vi "Config Unflatten.vi"(8 "error in (no error)":errorcluster, 10 "Raw Config":string, 11 "launcher in":refnum<class "launcher.lvclass">) -> (0 "error out":errorcluster, 1 "Modified?":bool, 3 "launcher out":refnum<class "launcher.lvclass">)   [LabVIEW 2021, in "launcher.lvclass"]
uses:
  launcher.lvclass
  launcher.lvclass/launcher.ctl
  5cad098a-3cfd-4683-b1d7-f77832a71d5c.vi
  9da31e51-d9e1-4e00-992a-b5057d501661.vi
  c0ef7aaf-9b39-40b0-914c-f7984f3f44cf.vi
  b278cc91-79ab-40b4-b454-5ce35c9e2d2c.vi
  Accessors/Read _PARMS.vi
  Accessors/Write _PARMS.vi
  <vilib>/JDP Science/JSONtext/JSON text to Variant.vi
  <vilib>/JDP Science/JSONtext/LVClass Serializer/JSONtext LVClass Serializer.lvclass
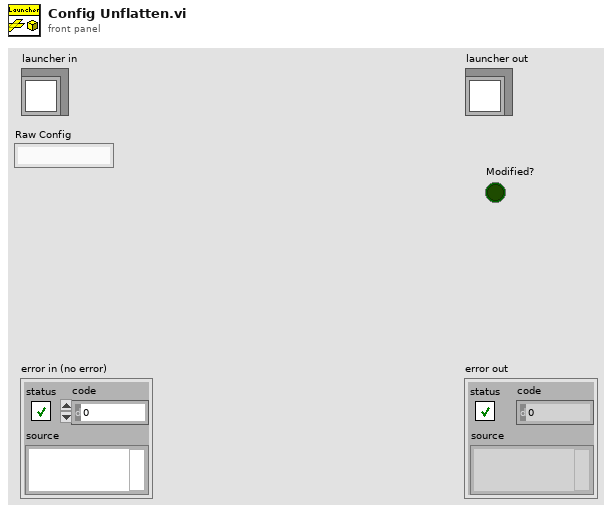
[diagram p1: front panel]
types:
  T1 = typedef "launcher.lvclass/_PARMS.ctl" = cluster{"ch_alias":string[], "ch_units":string[], "Modules to Launch":T2[]}
  T2 = typedef "Module.lvclass/Launch Module Typdef.ctl" = cluster{"Module":string, "Parameters":T3}
  T3 = typedef "Module.lvclass/Launch Module Parms.ctl" = cluster{"Name":string, "Arguments":string[], "Show FP?":bool}
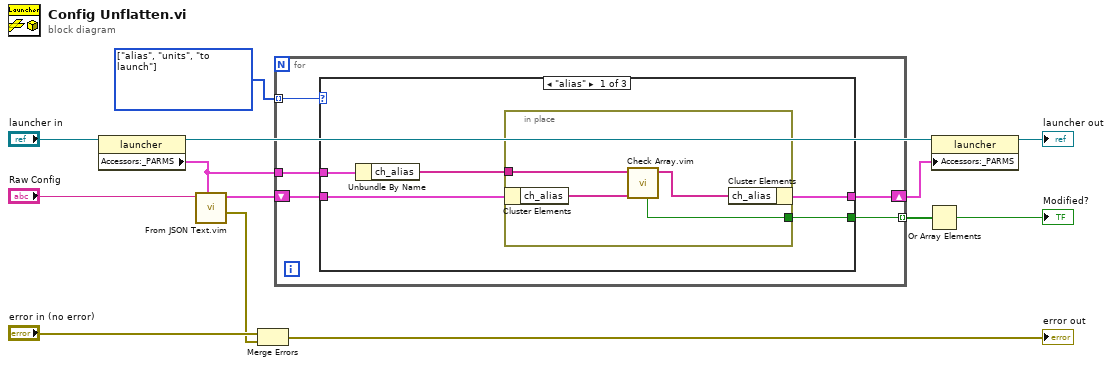
[diagram p0: block diagram]
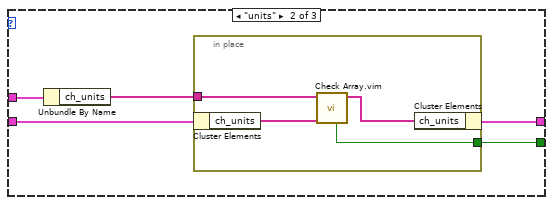
[diagram p2: hidden frame]
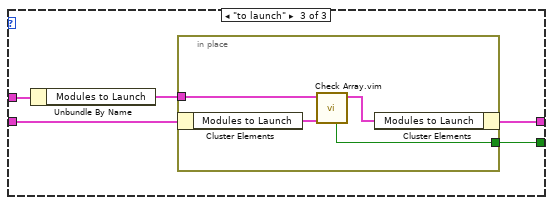
[diagram p3: hidden frame]
diagram:
  w7 = enum16{"alias", "units", "to launch"}[] [enum."alias", enum."units", enum."to launch"] items=["alias", "units", "to launch"]
  n1 = property class="launcher"(reference="launcher in") -> (reference out=w3:refnum<class "launcher.lvclass">, "Accessors:_PARMS"=w5:T1)  [unwired: 1 in, 1 out]
  n2 = call "From JSON Text.vim"("Data Type and Default Value"=w5, "JSON"="Raw Config") -> ("error out"=w9:errorcluster, "Data out"=w8:T1)  [unwired: 8 in]
  n3 = Merge Errors("error in (no error)", w9) -> (→"error out":errorcluster)
  n4 = for {
    shift-right: [w14] -> w2
    shift-left: w8 -> [w16]
    tunnel: w7 -> [w18] mode=indexing
    tunnel: w5 -> [w17]
    tunnel: [w15] -> w6 mode=indexing
    n5 = case shown="\"alias\"" w18 {
      tunnel: w17 -> [w22 w31 w40]
      tunnel: w16 -> [w21 w30 w39]
      tunnel: [w23 w32 w41] -> w15
      tunnel: [w19 w28 w37] -> w14
      frame "alias" {
        n6 = Unbundle By Name(w22) -> ("ch_alias"=w20:string[])
        n7 = in-place {
          in-place-border: [w26] -> w23
          in-place-border: w20 -> [w24]
          n8 = in-place-cluster #1(w21) -> ("ch_alias"=w25:string[])
          n9 = call "Check Array.vim"("Value in"=w25, "Default Value"=w24) -> ("Value out"=w27:string[], "Modified?"=w26:bool)  [unwired: 8 in]
          n10 = in-place-cluster #1("ch_alias"=w27) -> (w19:T1)
        }
      }
      frame "units" {
        n11 = Unbundle By Name(w31) -> ("ch_units"=w29:string[])
        n12 = in-place {
          in-place-border: [w35] -> w32
          in-place-border: w29 -> [w33]
          n13 = in-place-cluster #2(w30) -> ("ch_units"=w34:string[])
          n14 = call "Check Array.vim"("Value in"=w34, "Default Value"=w33) -> ("Value out"=w36:string[], "Modified?"=w35:bool)  [unwired: 8 in]
          n15 = in-place-cluster #2("ch_units"=w36) -> (w28:T1)
        }
      }
      frame "to launch" {
        n16 = Unbundle By Name(w40) -> ("Modules to Launch"=w38:T2[])
        n17 = in-place {
          in-place-border: [w44] -> w41
          in-place-border: w38 -> [w42]
          n18 = in-place-cluster #3(w39) -> ("Modules to Launch"=w43:T2[])
          n19 = call "Check Array.vim"("Value in"=w43, "Default Value"=w42) -> ("Value out"=w45:T2[], "Modified?"=w44:bool)  [unwired: 8 in]
          n20 = in-place-cluster #3("Modules to Launch"=w45) -> (w37:T1)
        }
      }
    }
  }
  n21 = Or Array Elements(Boolean array=w6) -> (logical OR=→"Modified?":bool)
  n22 = property class="launcher"(reference=w3, "Accessors:_PARMS"=w2) -> (reference out=→"launcher out":refnum<class "launcher.lvclass">)  [unwired: 1 in, 1 out]
